vi "ManualOverrideOCU.vi"() -> ()   [LabVIEW 2011]
uses:
  2-RIO/2 Typedefs/manual override.ctl
  2-RIO/2 Typedefs/setpoints to boat.ctl
  2-RIO/2 Typedefs/sail setpt.ctl
  2-RIO/2 Typedefs/rudder angle.ctl
  <vilib>/Utility/inputDevices.llb/closeKeyboard.vi
  2-RIO/2 Globals/2 Global.vi
  <vilib>/Utility/inputDevices.llb/keyboardAcquire.vi
panel:
  out "Manual Override Cluster":T1
  in  "OVERRIDE?":bool
  out "keys pressed":T5(array[ring])
  out "Rudder":dbl
  out "Sails":dbl
  in  "VI stop":bool
  in  "Full Port":bool
  in  "Port":bool
  in  "Full Starboard":bool
  in  "Starboard":bool
  out "Sent Rudder Angle":dbl(slide) scale=250.0..50.0
  out "Sent Sail In/Out Value":dbl(slide) scale=250.0..50.0
  in  "Full In":bool
  in  "Sheet In":bool
  in  "Full Out":bool
  in  "Sheet Out":bool
  # "This is the Manual Override OCU:\nMake a manual override interface that can be added to the OCU (complete with keyboard control), and a typedef for the data the interface outputs. Make a separate VI that inputs data with this typedef and uses it to actually control the small RC boat. Use the system diagram (in 'required documentation' below) for reference.\nCommit code to the appropriate folders on the SVN repository."
  # "SAIL CONTROL"
  # "OUT = 90"
  # "UP"
  # "IN = 210"
  # "DOWN"
  # "RUDDER CONTROL"
  # "PORT = 210"
  # "STARB = 90"
  # "LEFT"
  # "RIGHT"
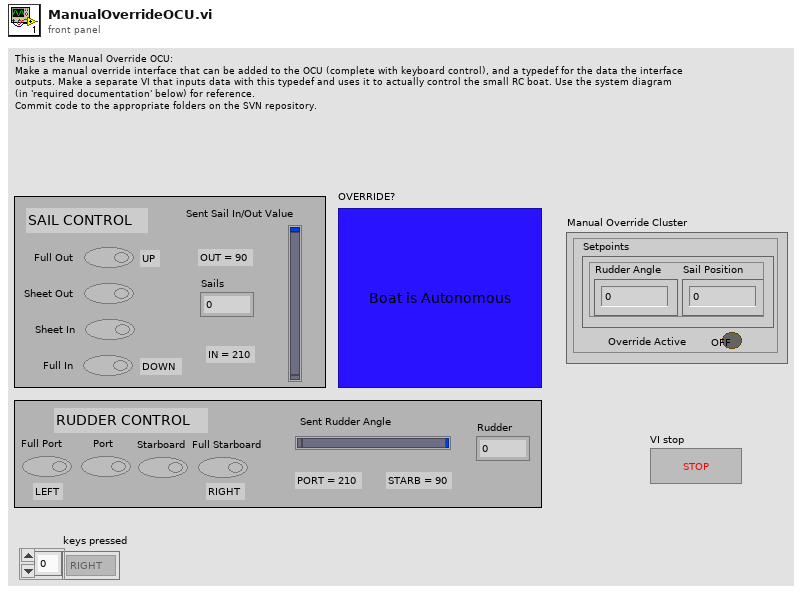
[diagram p1: front panel]
types:
  T1 = typedef "manual override.ctl" = cluster{"Override Active":bool, "Setpoints":T2}
  T2 = typedef "setpoints to boat.ctl" = cluster{"Sail Position":T3, "Rudder Angle":T4}
  T3 = typedef "sail setpt.ctl" = dbl
  T4 = typedef "rudder angle.ctl" = dbl
  T5 = enum16{"0", "1", "2", "3", "4", "5", "6", "7", "8", "9", "A", "B", "C", "D", "E", "F", "G", "H", "I", "J", "K", "L", "M", "N", "O", "P", "Q", "R", "S", "T", "U", "V", "W", "X", "Y", "Z", "F1", "F2", "F3", "F4", "F5", "F6", "F7", "F8", "F9", "F10", "F11", "F12", "F13", "F14", "F15", "ADD", "BACK", "BACKSLASH", "CAPITAL", "COMMA", "DECIMAL", "DELETE", "DIVIDE", "DOWN", "END", "EQUALS", "ESCAPE", "GRAVE (`)", "HOME", "INSERT", "LBRACKET", "LCONTROL", "LEFT", "L ALT", "LSHIFT", "LWIN", "MINUS", "MULTIPLY", "NEXT", "NUMLOCK", "NUMPAD_0", "NUMPAD_1", "NUMPAD_2", "NUMPAD_3", "NUMPAD_4", "NUMPAD_5", "NUMPAD_6", "NUMPAD_7", "NUMPAD_8", "NUMPAD_9", "PAUSE", "PERIOD", "PRIOR (PG UP)", "RBRACKET", "RCONTROL", "RETURN", "RIGHT", "R ALT", "RSHIFT", "RWIN", "SCROLL", "SEMICOLON", "SLASH", "SPACE", "SUBTRACT", "TAB", "UP", "ENTER (num pad)", "' (quote)"}[]
  T6 = enum16{"0", "1", "2", "3", "4", "5", "6", "7", "8", "9", "A", "B", "C", "D", "E", "F", "G", "H", "I", "J", "K", "L", "M", "N", "O", "P", "Q", "R", "S", "T", "U", "V", "W", "X", "Y", "Z", "F1", "F2", "F3", "F4", "F5", "F6", "F7", "F8", "F9", "F10", "F11", "F12", "F13", "F14", "F15", "ADD", "BACK", "BACKSLASH", "CAPITAL", "COMMA", "DECIMAL", "DELETE", "DIVIDE", "DOWN", "END", "EQUALS", "ESCAPE", "GRAVE (`)", "HOME", "INSERT", "LBRACKET", "LCONTROL", "LEFT", "L ALT", "LSHIFT", "LWIN", "MINUS", "MULTIPLY", "NEXT", "NUMLOCK", "NUMPAD_0", "NUMPAD_1", "NUMPAD_2", "NUMPAD_3", "NUMPAD_4", "NUMPAD_5", "NUMPAD_6", "NUMPAD_7", "NUMPAD_8", "NUMPAD_9", "PAUSE", "PERIOD", "PRIOR (PG UP)", "RBRACKET", "RCONTROL", "RETURN", "RIGHT", "R ALT", "RSHIFT", "RWIN", "SCROLL", "SEMICOLON", "SLASH", "SPACE", "SUBTRACT", "TAB", "UP", "ENTER (num pad)", "' (quote)"}
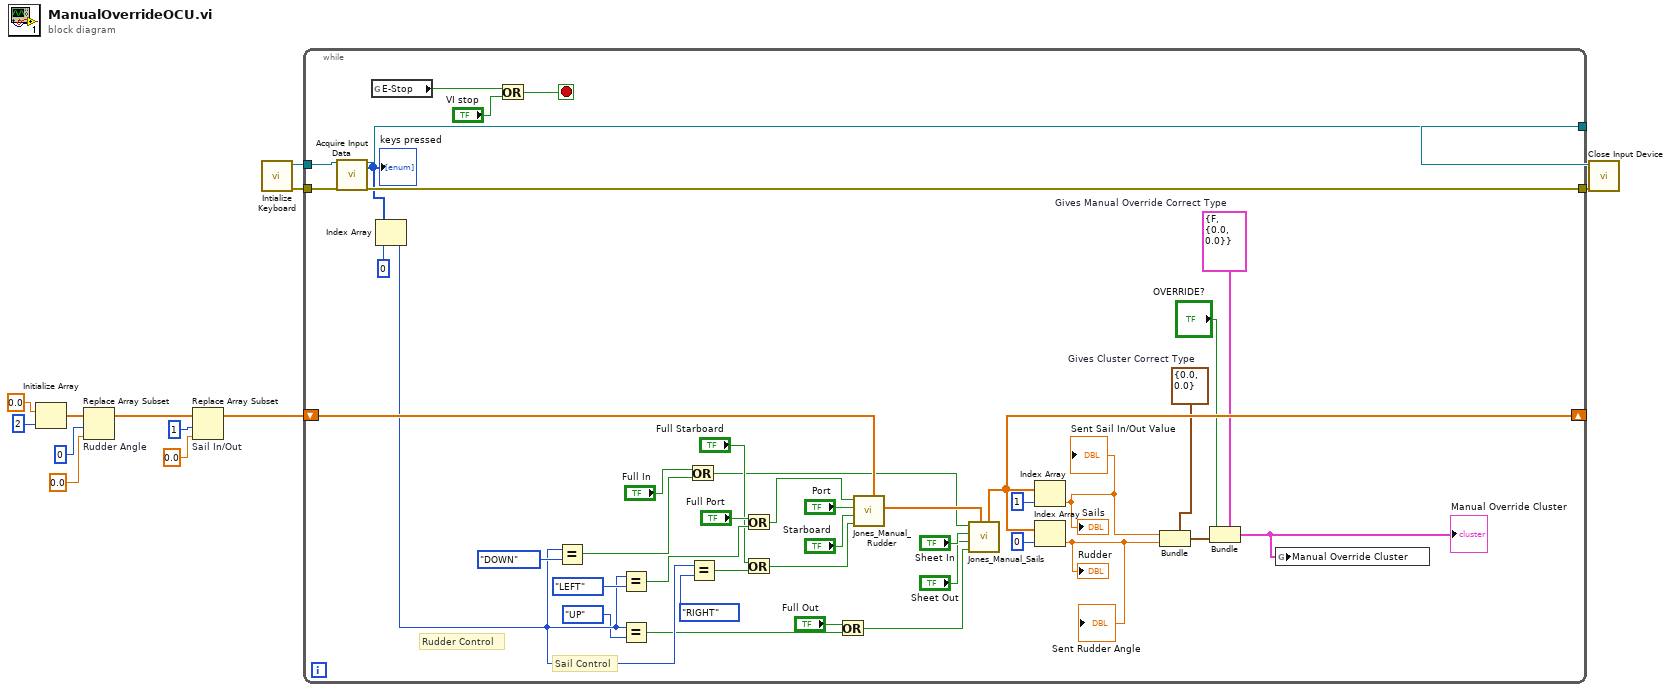
[diagram p0: block diagram]
diagram:
  n1 = Initialize Array(0.0 ("element"), 2 ("dimension size")) -> (w4:dbl[])
  n2 = Replace Array Subset "Rudder Angle"(array=w4, new element=0.0 ("new element/subarray"), index=0) -> (w6:dbl[])
  n3 = Replace Array Subset "Sail In/Out"(array=w6, new element=0.0 ("new element/subarray"), index=1) -> (w3:dbl[])
  n4 = call <vilib>:"Intialize Keyboard.vi"() -> ("error out"=w13:errorcluster, "device ID"=w12:refnum<k1>)  [unwired: 10 in]
  n5 = while {
    shift-right: [w23] -> _
    shift-left: w3 -> [w44]
    tunnel: w13 -> [w52]
    tunnel: w12 -> [w51]
    tunnel: [w50] -> w11
    tunnel: [w49] -> w10
    stop <- w17 stop-if-true
    w14 = T2 {"Sail Position"=0.0, "Rudder Angle"=0.0}  # Gives Cluster Correct Type
    w15 = T1 {"Override Active"=FALSE, "Setpoints"={"Sail Position"=0.0, "Rudder Angle"=0.0}}  # Gives Manual Override Correct Type
    # "Sail Control"
    # "Rudder Control"
    n6 = call-poly <vilib>:"Acquire Input Data.vi"("device ID"=w51, "error in (no error)"=w52) -> ("device ID"=w50:refnum<k1>, "keys pressed"=w48:T5, "error out"=w49:errorcluster)  [unwired: 15 in]
    "keys pressed" <- w48
    n7 = global read "2 Global.vi" "E-Stop"() -> (w16:bool)
    n8 = Index Array(array=w48, index=0) -> (element=w28:T6)
    n9 = Or(x=w16, y="VI stop") -> (x .or. y?=w17:bool)
    n10 = Equal?(x=w28, y=T6."DOWN" ("element 2")) -> (x = y?=w31:bool)
    n11 = Equal?(x=w28, y=T6."LEFT" ("element 2")) -> (x = y?=w39:bool)
    n12 = Equal?(x=w28, y=T6."UP" ("element 2")) -> (x = y?=w26:bool)
    n13 = Or(x="Full In", y=w31) -> (x .or. y?=w30:bool)
    n14 = Equal?(x=w28, y=T6."RIGHT" ("element 2")) -> (x = y?=w34:bool)
    n15 = Or(x="Full Port", y=w39) -> (x .or. y?=w37:bool)
    n16 = Or(x="Full Starboard", y=w34) -> (x .or. y?=w35:bool)
    n17 = Or(x="Full Out", y=w26) -> (x .or. y?=w24:bool)
    n18 = call "Jones_Manual_Rudder.vi"("Full Port"=w37, "Port"="Port", "Starboard"="Starboard", "Full Starboard"=w35, "Array"=w44) -> ("Array 2"=w41:dbl[])  [unwired: 3 in]
    n19 = call "Jones_Manual_Sails.vi"("Full In"=w30, "Sheet In"="Sheet In", "Sheet Out"="Sheet Out", "Full Out"=w24, "Array"=w41) -> ("Array 2"=w23:dbl[])  [unwired: 5 in]
    n20 = Index Array(array=w23, index=1) -> (element=w21:dbl)
    "Sent Sail In/Out Value" <- w21
    "Sails" <- w21
    n21 = Index Array(array=w23, index=0) -> (element=w22:dbl)
    "Sent Rudder Angle" <- w22
    "Rudder" <- w22
    n22 = Bundle(cluster=w14, "Sail Position"=w21, "Rudder Angle"=w22) -> (w20:T2)
    n23 = Bundle(cluster=w15, "Override Active"="OVERRIDE?", "Setpoints"=w20) -> (w18:T1)
    "Manual Override Cluster" <- w18
    n24 = global write "2 Global.vi" "Manual Override Cluster"(w18) -> ()
  }
  n25 = call-poly <vilib>:"Close Input Device.vi"("error in (no error)"=w10, "device ID"=w11) -> ()  [unwired: 8 in, 1 out]
